vi "Lian_Charts_and_Graphs.vi"() -> ()   [LabVIEW 2020]
uses:
  <vilib>/measure/NI_MABase.lvlib
panel:
  out "Waveform Chart 6":waveform(dbl)(graph)={"t0"=timestamp(13.0 s since 1904-01-01), "dt"=0.001, "Y"=array[1000 elements]}
  out "Waveform Chart 5":waveform(dbl)(graph)={"t0"=timestamp(13.0 s since 1904-01-01), "dt"=0.001, "Y"=array[1000 elements]}
  out "Waveform Chart 4":waveform(dbl)(graph)={"t0"=timestamp(13.0 s since 1904-01-01), "dt"=0.001, "Y"=array[1000 elements]}
  out "Waveform Chart 3":waveform(dbl)(graph)={"t0"=timestamp(13.0 s since 1904-01-01), "dt"=0.001, "Y"=array[1000 elements]}
  out "Waveform Chart 2":waveform(dbl)(graph)={"t0"=timestamp(13.0 s since 1904-01-01), "dt"=0.001, "Y"=array[1000 elements]}
  out "Waveform Chart 1":waveform(dbl)(graph)={"t0"=timestamp(13.0 s since 1904-01-01), "dt"=0.001, "Y"=array[1000 elements]}
  in  "Loop Delay (ms)":u32=1000
  in  "offset":dbl format="%0.2p"
  in  "square wave duty cycle (%)":dbl=50.0 format="%0.2f"
  in  "sampling info":cluster{"Fs":dbl, "#s":dbl}={"Fs"=1000.0, "#s"=1000.0} {"Fs" format="%.2p"}
  in  "phase":dbl format="%.2p"
  in  "amplitude":dbl=4.0 format="%0.2p"
  in  "frequency":dbl=10.0 format="%0.2p"
  in  "signal type":T1(ring)
  in  "stop":bool
  # "Waveform Generation"
  # "Waveform Charts"
  # "Absolute Time - Default Timestamp"
  # "Relative Time"
  # "Absolute Time - Updated Timestamp"
  # "Scope Chart"
  # "Floating Point"
  # "Sweep Chart"
  # "Loop Timing"
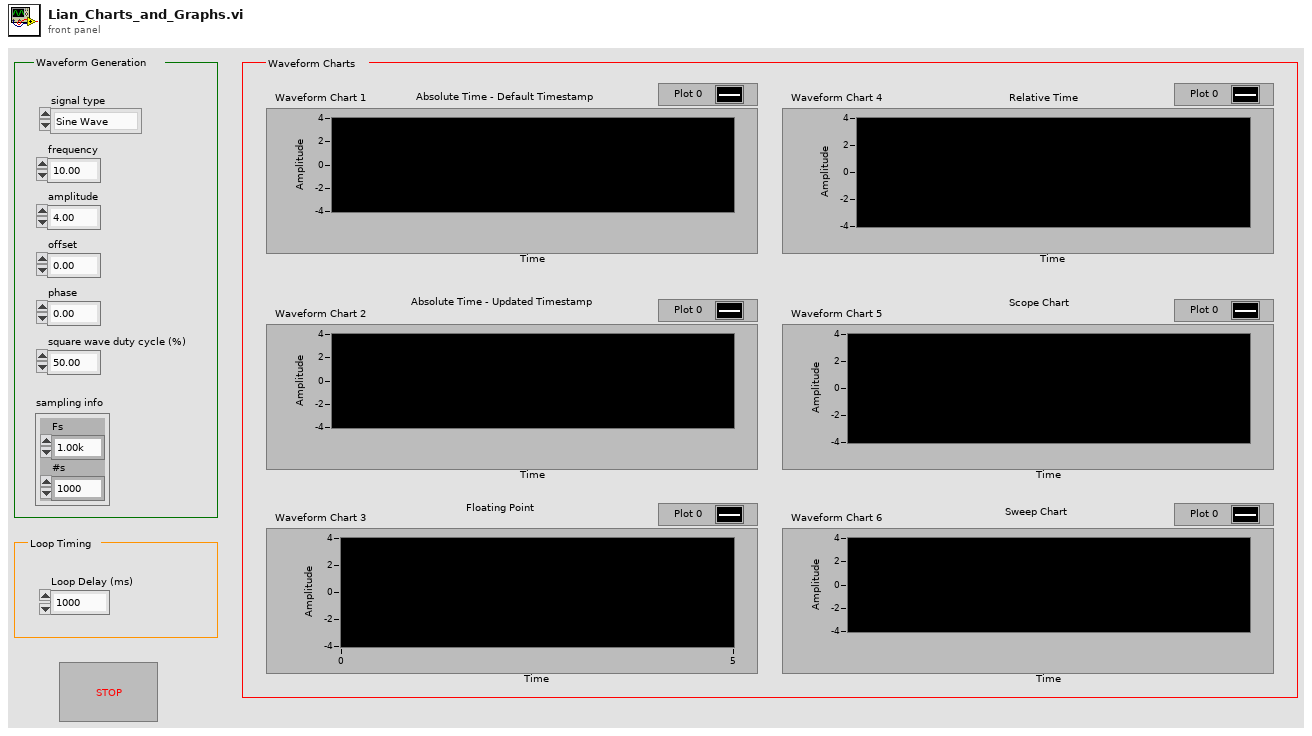
[diagram p1: front panel]
types:
  T1 = enum16{"Sine Wave", "Triangle Wave", "Square Wave", "Sawtooth Wave"}
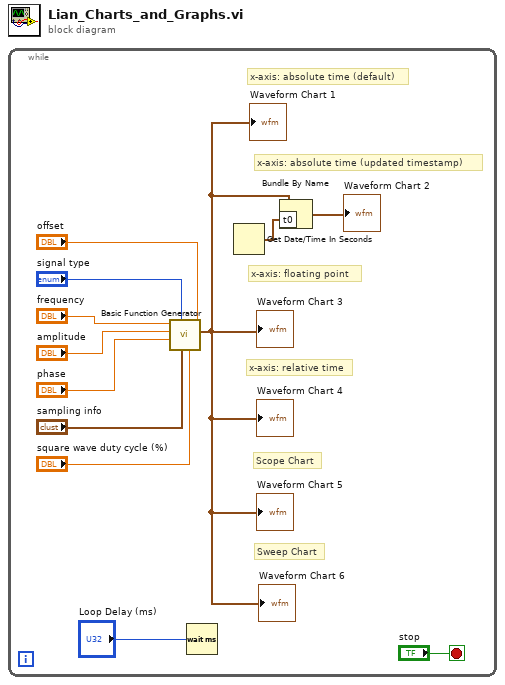
[diagram p0: block diagram]
diagram:
  n1 = while {
    stop <- "stop" stop-if-true
    # "x-axis: floating point"
    # "x-axis: absolute time (default)"
    # "Sweep Chart"
    # "Scope Chart"
    # "x-axis: absolute time (updated timestamp)"
    # "x-axis: relative time"
    n2 = call <vilib>:"Basic Function Generator.vi"("offset"="offset", "square wave duty cycle (%)"="square wave duty cycle (%)", "sampling info"="sampling info", "signal type"="signal type", "phase"="phase", "amplitude"="amplitude", "frequency"="frequency") -> ("signal out"=w1:waveform(dbl))  [unwired: 2 in, 2 out]
    "Waveform Chart 1" <- w1
    "Waveform Chart 3" <- w1
    "Waveform Chart 4" <- w1
    "Waveform Chart 5" <- w1
    "Waveform Chart 6" <- w1
    n3 = Wait (ms)(milliseconds to wait="Loop Delay (ms)") -> ()  [unwired: 1 out]
    n4 = Get Date/Time In Seconds() -> (seconds since 1Jan1904=w3:timestamp)
    n5 = Bundle By Name(cluster=w1, "t0"=w3) -> (→"Waveform Chart 2":waveform(dbl))
  }
